vi "_CSMObj-Release.vi"(8 "Error in":errorcluster caption="Error in (no error)", 11 "CSMQ in":T1={"Requested Name"="", "Module Name"="", "Mode"=enum."Stand Alone", "Queue"=refnum, "CSM-Data"=refnum, "User Event"=refnum, "Status Change Event"=refnum, "Allowed Messages"=[], "Mode-Data"=refnum, "Group Name"="", "Exit Event"=refnum}) -> (0 "Error out":errorcluster, 1 "Group Release?":bool, 3 "CSMQ out":T1={"Requested Name"="", "Module Name"="", "Mode"=enum."Stand Alone", "Queue"=refnum, "CSM-Data"=refnum, "User Event"=refnum, "Status Change Event"=refnum, "Allowed Messages"=[], "Mode-Data"=refnum, "Group Name"="", "Exit Event"=refnum})   [LabVIEW 2020, in "Communicable State Machine.lvlib"]
uses:
  Communicable State Machine.lvlib
  _CSMObj.ctl
  Priority Queue.lvclass
  _CSM_MODE.ctl
  _CSMObj-Data.ctl
  _CSM Status Change Event Data.ctl
  _CSMObj-ModeData.ctl
  Priority Queue.lvclass/Priority Queue.ctl
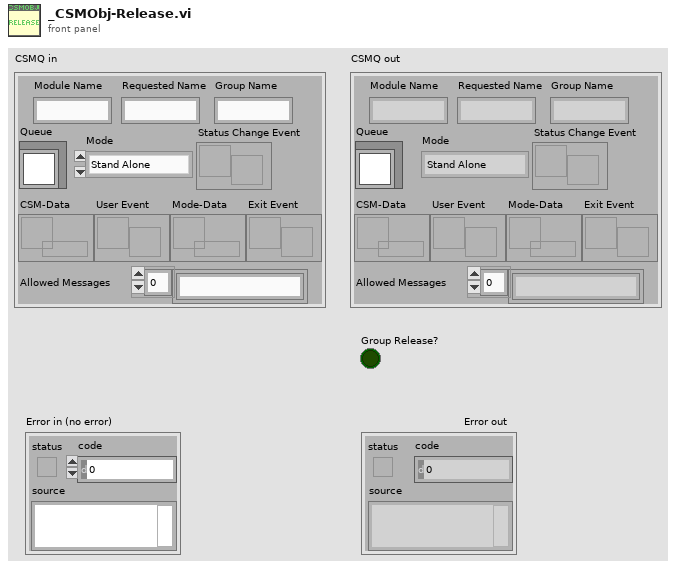
[diagram p1: front panel]
types:
  T1 = typedef "Communicable State Machine.lvlib/_CSMObj.ctl" = cluster{"Requested Name":string, "Module Name":string, "Mode":T2, "Queue":refnum<class "Priority Queue.lvclass">, "CSM-Data":refnum<data-value>, "User Event":refnum<user-event>, "Status Change Event":refnum<user-event>, "Allowed Messages":string[], "Mode-Data":refnum<data-value>, "Group Name":string, "Exit Event":refnum<user-event>}
  T2 = typedef "Communicable State Machine.lvlib/_CSM_MODE.ctl" = enum16{"Not Exist", "Stand Alone", "CSM", "Worker Agent", "Worker", "Chain", "Chain Node"}
  T3 = typedef "Communicable State Machine.lvlib/_CSMObj-ModeData.ctl" = cluster{"Share Count":i32, "Messages of Chain Nodes":cluster{"Module Name":string, "Allowed Messages":string[]}[], "Chain Message Mapping Map":variant}
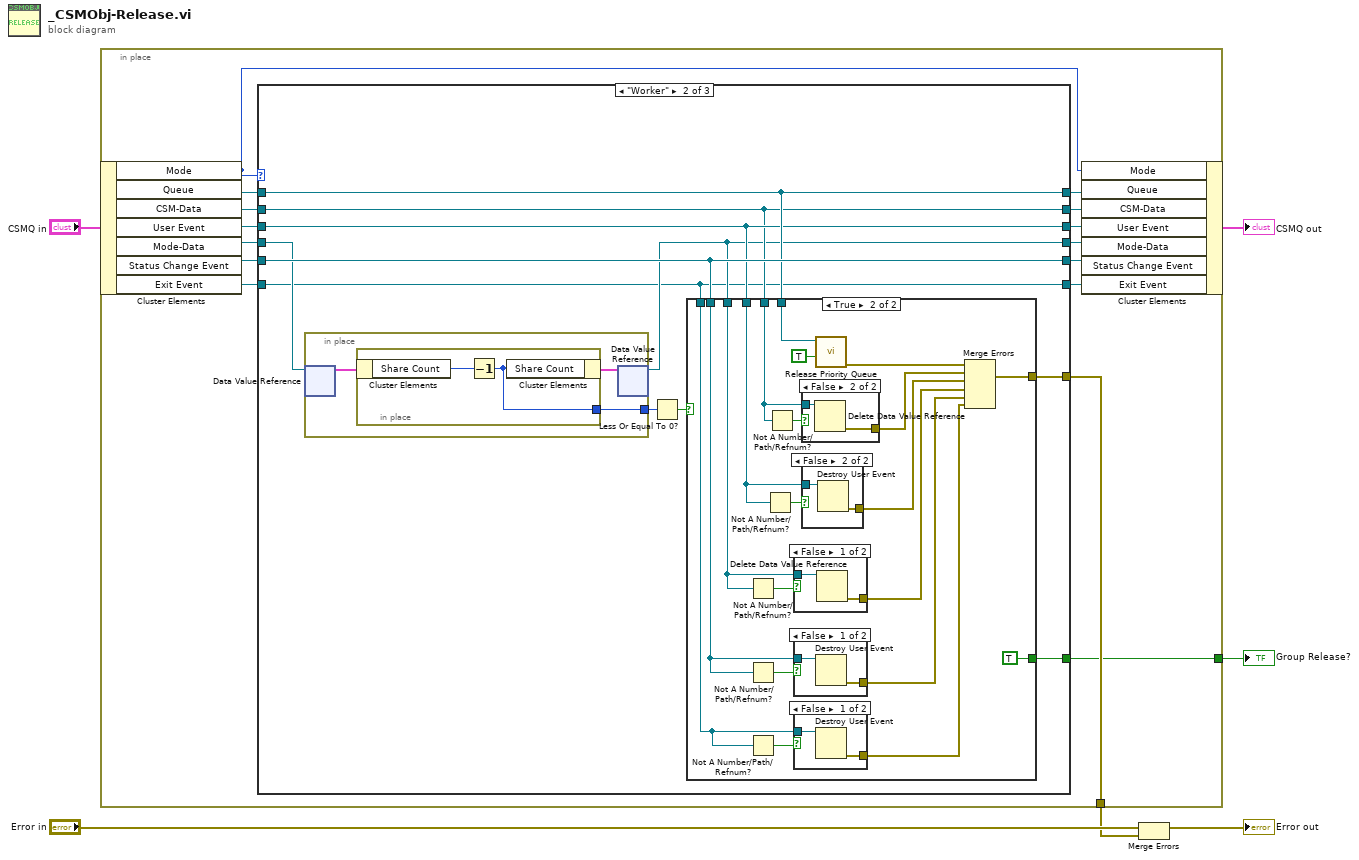
[diagram p0: block diagram]
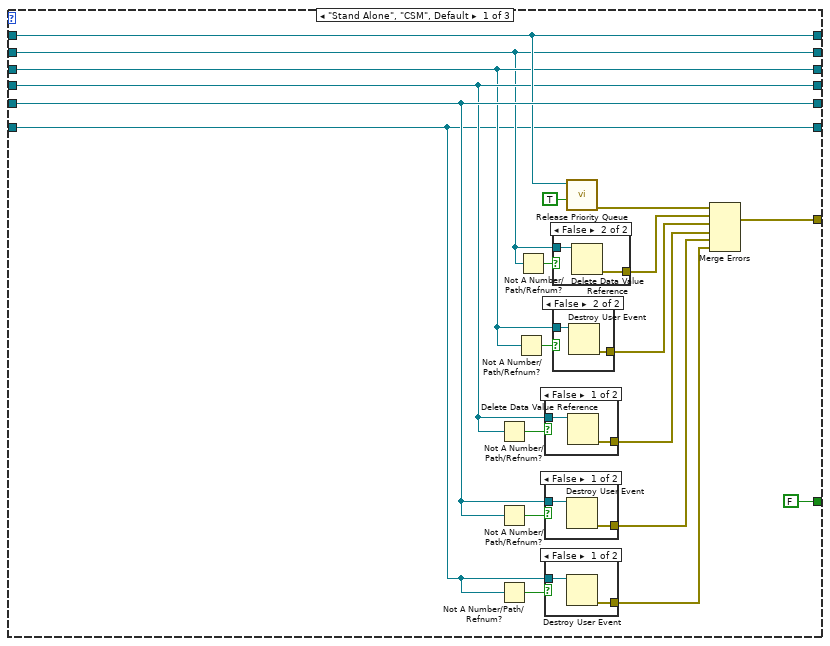
[diagram p2: hidden frame]
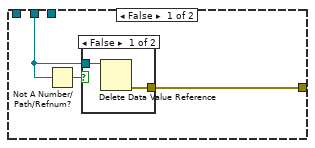
[diagram p8: hidden frame]
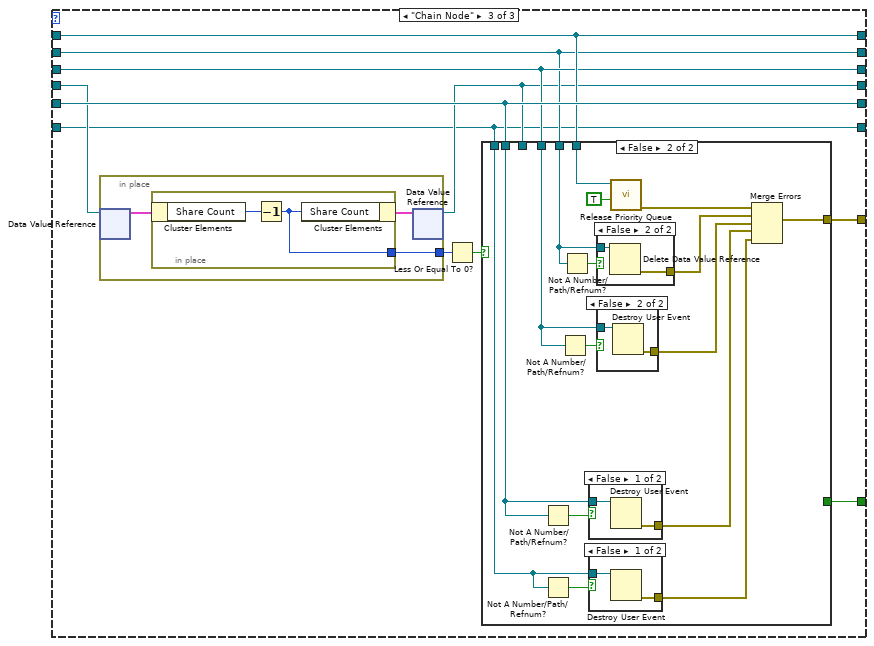
[diagram p15: hidden frame]
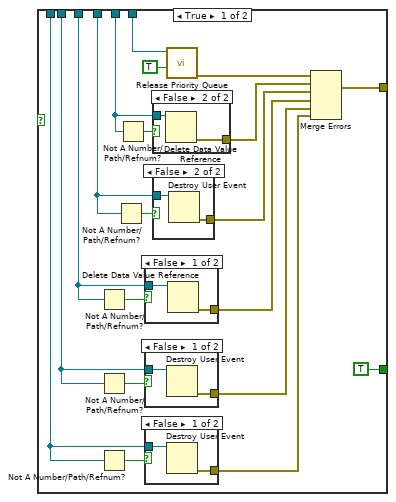
[diagram p16: hidden frame]
diagram:
  n1 = in-place "In Place Element Structure" {
    in-place-border: [w12] -> w2
    in-place-border: [w11] -> w1
    n2 = in-place-cluster #1("CSMQ in") -> ("Mode"=w9:T2, "Queue"=w17:refnum<class "Priority Queue.lvclass">, "CSM-Data"=w20:refnum<data-value>, "User Event"=w19:refnum<user-event>, "Mode-Data"=w21:refnum<data-value>, "Status Change Event"=w18:refnum<user-event>, "Exit Event"=w7:refnum<user-event>)
    n3 = case shown="\"Worker\"" w9 {
      tunnel: w21 -> [w29 w56 w107]
      tunnel: w20 -> [w26 w57 w108]
      tunnel: w19 -> [w28 w58 w109]
      tunnel: w18 -> [w41 w62 w113]
      tunnel: w17 -> [w40 w61 w112]
      tunnel: [w41 w62 w113] -> w16
      tunnel: [w28 w58 w109] -> w15
      tunnel: [w26 w57 w108] -> w14
      tunnel: [w40 w61 w112] -> w13
      tunnel: [w39 w60 w111] -> w12
      tunnel: [FALSE w59 w110] -> w11
      tunnel: [w29 w55 w106] -> w10
      tunnel: [w23 w52 w103] -> w8
      tunnel: w7 -> [w23 w52 w103]
      frame "Stand Alone", "CSM", Default {
        n4 = Not A Number/Path/Refnum?(number/path/refnum=w29) -> (NaN/Path/Refnum?=w31:bool)
        n5 = Not A Number/Path/Refnum?(number/path/refnum=w41) -> (NaN/Path/Refnum?=w32:bool)
        n6 = Not A Number/Path/Refnum?(number/path/refnum=w23) -> (NaN/Path/Refnum?=w24:bool)
        n7 = Not A Number/Path/Refnum?(number/path/refnum=w28) -> (NaN/Path/Refnum?=w27:bool)
        n8 = Not A Number/Path/Refnum?(number/path/refnum=w26) -> (NaN/Path/Refnum?=w25:bool)
        n9 = case shown="False" w31 {
          tunnel: [w49 _] -> w30
          tunnel: w29 -> [w48 _]
          frame False {
            n10 = Delete Data Value Reference(data value reference=w48) -> (error out=w49:errorcluster)  [unwired: 1 in, 1 out]
          }
          frame True {
          }
        }
        n11 = case shown="False" w32 {
          tunnel: [w51 _] -> w33
          tunnel: w41 -> [w50 _]
          frame False {
            n12 = Destroy User Event(user event=w50) -> (error out=w51:errorcluster)  [unwired: 1 in]
          }
          frame True {
          }
        }
        n13 = case shown="False" w24 {
          tunnel: [w43 _] -> w22
          tunnel: w23 -> [w42 _]
          frame False {
            n14 = Destroy User Event(user event=w42) -> (error out=w43:errorcluster)  [unwired: 1 in]
          }
          frame True {
          }
        }
        n15 = case shown="False" w25 {
          tunnel: [_ w45] -> w35
          tunnel: w26 -> [_ w44]
          frame True {
          }
          frame False {
            n16 = Delete Data Value Reference(data value reference=w44) -> (error out=w45:errorcluster)  [unwired: 1 in, 1 out]
          }
        }
        n17 = case shown="False" w27 {
          tunnel: [_ w47] -> w34
          tunnel: w28 -> [_ w46]
          frame True {
          }
          frame False {
            n18 = Destroy User Event(user event=w46) -> (error out=w47:errorcluster)  [unwired: 1 in]
          }
        }
        n19 = call "Release Priority Queue.vi"("force destroy? (F)"=TRUE, "Priority Queue"=w40) -> ("error out"=w36:errorcluster)  [unwired: 9 in]
        n20 = Merge Errors(w36, w35, w34, w30, w33, w22) -> (w39:errorcluster)
      }
      frame "Worker" {
        n21 = in-place {
          in-place-border: [w98] -> w54
          n22 = in-place-dvr #2(w56) -> (w100:T3)  [unwired: 1 out]
          n23 = in-place {
            in-place-border: [w101] -> w98
            n24 = in-place-cluster #3(w100) -> ("Share Count"=w102:i32)
            n25 = Decrement(x=w102) -> (x-1=w101:i32)
            n26 = in-place-cluster #3("Share Count"=w101) -> (w99:T3)
          }
          n27 = in-place-dvr #2(w99) -> (w55:refnum<data-value>)  [unwired: 1 out]
        }
        n28 = Less Or Equal To 0?(x=w54) -> (x <= 0?=w53:bool)
        n29 = case shown="True" w53 {
          tunnel: w62 -> [_ w87]
          tunnel: w61 -> [_ w86]
          tunnel: [w63 w85] -> w60
          tunnel: [_ TRUE] -> w59
          tunnel: w58 -> [_ w75]
          tunnel: w57 -> [w64 w73]
          tunnel: w55 -> [_ w71]
          tunnel: w52 -> [_ w69]
          frame False {
            n30 = Not A Number/Path/Refnum?(number/path/refnum=w64) -> (NaN/Path/Refnum?=w65:bool)
            n31 = case shown="False" w65 {
              tunnel: [w67 _] -> w63
              tunnel: w64 -> [w66 _]
              frame False {
                n32 = Delete Data Value Reference(data value reference=w66) -> (error out=w67:errorcluster)  [unwired: 1 in, 1 out]
              }
              frame True {
              }
            }
          }
          frame True {
            n33 = Not A Number/Path/Refnum?(number/path/refnum=w71) -> (NaN/Path/Refnum?=w77:bool)
            n34 = Not A Number/Path/Refnum?(number/path/refnum=w87) -> (NaN/Path/Refnum?=w78:bool)
            n35 = Not A Number/Path/Refnum?(number/path/refnum=w69) -> (NaN/Path/Refnum?=w70:bool)
            n36 = Not A Number/Path/Refnum?(number/path/refnum=w75) -> (NaN/Path/Refnum?=w74:bool)
            n37 = Not A Number/Path/Refnum?(number/path/refnum=w73) -> (NaN/Path/Refnum?=w72:bool)
            n38 = case shown="False" w77 {
              tunnel: [w95 _] -> w76
              tunnel: w71 -> [w94 _]
              frame False {
                n39 = Delete Data Value Reference(data value reference=w94) -> (error out=w95:errorcluster)  [unwired: 1 in, 1 out]
              }
              frame True {
              }
            }
            n40 = case shown="False" w78 {
              tunnel: [w97 _] -> w79
              tunnel: w87 -> [w96 _]
              frame False {
                n41 = Destroy User Event(user event=w96) -> (error out=w97:errorcluster)  [unwired: 1 in]
              }
              frame True {
              }
            }
            n42 = case shown="False" w70 {
              tunnel: [w89 _] -> w68
              tunnel: w69 -> [w88 _]
              frame False {
                n43 = Destroy User Event(user event=w88) -> (error out=w89:errorcluster)  [unwired: 1 in]
              }
              frame True {
              }
            }
            n44 = case shown="False" w72 {
              tunnel: [_ w91] -> w81
              tunnel: w73 -> [_ w90]
              frame True {
              }
              frame False {
                n45 = Delete Data Value Reference(data value reference=w90) -> (error out=w91:errorcluster)  [unwired: 1 in, 1 out]
              }
            }
            n46 = case shown="False" w74 {
              tunnel: [_ w93] -> w80
              tunnel: w75 -> [_ w92]
              frame True {
              }
              frame False {
                n47 = Destroy User Event(user event=w92) -> (error out=w93:errorcluster)  [unwired: 1 in]
              }
            }
            n48 = call "Release Priority Queue.vi"("force destroy? (F)"=TRUE, "Priority Queue"=w86) -> ("error out"=w82:errorcluster)  [unwired: 9 in]
            n49 = Merge Errors(w82, w81, w80, w76, w79, w68) -> (w85:errorcluster)
          }
        }
      }
      frame "Chain Node" {
        n50 = in-place {
          in-place-border: [w168] -> w105
          n51 = in-place-dvr #4(w107) -> (w170:T3)  [unwired: 1 out]
          n52 = in-place {
            in-place-border: [w171] -> w168
            n53 = in-place-cluster #5(w170) -> ("Share Count"=w172:i32)
            n54 = Decrement(x=w172) -> (x-1=w171:i32)
            n55 = in-place-cluster #5("Share Count"=w171) -> (w169:T3)
          }
          n56 = in-place-dvr #4(w169) -> (w106:refnum<data-value>)  [unwired: 1 out]
        }
        n57 = Less Or Equal To 0?(x=w105) -> (x <= 0?=w104:bool)
        n58 = case shown="False" w104 {
          tunnel: w113 -> [w133 w159]
          tunnel: w112 -> [w132 w158]
          tunnel: [w131 w157] -> w111
          tunnel: [TRUE _] -> w110
          tunnel: w109 -> [w121 w150]
          tunnel: w108 -> [w119 w148]
          tunnel: w106 -> [w117 _]
          tunnel: w103 -> [w115 w145]
          frame True {
            n59 = Not A Number/Path/Refnum?(number/path/refnum=w117) -> (NaN/Path/Refnum?=w123:bool)
            n60 = Not A Number/Path/Refnum?(number/path/refnum=w133) -> (NaN/Path/Refnum?=w124:bool)
            n61 = Not A Number/Path/Refnum?(number/path/refnum=w115) -> (NaN/Path/Refnum?=w116:bool)
            n62 = Not A Number/Path/Refnum?(number/path/refnum=w121) -> (NaN/Path/Refnum?=w120:bool)
            n63 = Not A Number/Path/Refnum?(number/path/refnum=w119) -> (NaN/Path/Refnum?=w118:bool)
            n64 = case shown="False" w123 {
              tunnel: [w141 _] -> w122
              tunnel: w117 -> [w140 _]
              frame False {
                n65 = Delete Data Value Reference(data value reference=w140) -> (error out=w141:errorcluster)  [unwired: 1 in, 1 out]
              }
              frame True {
              }
            }
            n66 = case shown="False" w124 {
              tunnel: [w143 _] -> w125
              tunnel: w133 -> [w142 _]
              frame False {
                n67 = Destroy User Event(user event=w142) -> (error out=w143:errorcluster)  [unwired: 1 in]
              }
              frame True {
              }
            }
            n68 = case shown="False" w116 {
              tunnel: [w135 _] -> w114
              tunnel: w115 -> [w134 _]
              frame False {
                n69 = Destroy User Event(user event=w134) -> (error out=w135:errorcluster)  [unwired: 1 in]
              }
              frame True {
              }
            }
            n70 = case shown="False" w118 {
              tunnel: [_ w137] -> w127
              tunnel: w119 -> [_ w136]
              frame True {
              }
              frame False {
                n71 = Delete Data Value Reference(data value reference=w136) -> (error out=w137:errorcluster)  [unwired: 1 in, 1 out]
              }
            }
            n72 = case shown="False" w120 {
              tunnel: [_ w139] -> w126
              tunnel: w121 -> [_ w138]
              frame True {
              }
              frame False {
                n73 = Destroy User Event(user event=w138) -> (error out=w139:errorcluster)  [unwired: 1 in]
              }
            }
            n74 = call "Release Priority Queue.vi"("force destroy? (F)"=TRUE, "Priority Queue"=w132) -> ("error out"=w128:errorcluster)  [unwired: 9 in]
            n75 = Merge Errors(w128, w127, w126, w122, w125, w114) -> (w131:errorcluster)
          }
          frame False {
            n76 = Not A Number/Path/Refnum?(number/path/refnum=w159) -> (NaN/Path/Refnum?=w151:bool)
            n77 = Not A Number/Path/Refnum?(number/path/refnum=w145) -> (NaN/Path/Refnum?=w146:bool)
            n78 = Not A Number/Path/Refnum?(number/path/refnum=w150) -> (NaN/Path/Refnum?=w149:bool)
            n79 = Not A Number/Path/Refnum?(number/path/refnum=w148) -> (NaN/Path/Refnum?=w147:bool)
            n80 = case shown="False" w151 {
              tunnel: [w167 _] -> w152
              tunnel: w159 -> [w166 _]
              frame False {
                n81 = Destroy User Event(user event=w166) -> (error out=w167:errorcluster)  [unwired: 1 in]
              }
              frame True {
              }
            }
            n82 = case shown="False" w146 {
              tunnel: [w161 _] -> w144
              tunnel: w145 -> [w160 _]
              frame False {
                n83 = Destroy User Event(user event=w160) -> (error out=w161:errorcluster)  [unwired: 1 in]
              }
              frame True {
              }
            }
            n84 = case shown="False" w147 {
              tunnel: [_ w163] -> w154
              tunnel: w148 -> [_ w162]
              frame True {
              }
              frame False {
                n85 = Delete Data Value Reference(data value reference=w162) -> (error out=w163:errorcluster)  [unwired: 1 in, 1 out]
              }
            }
            n86 = case shown="False" w149 {
              tunnel: [_ w165] -> w153
              tunnel: w150 -> [_ w164]
              frame True {
              }
              frame False {
                n87 = Destroy User Event(user event=w164) -> (error out=w165:errorcluster)  [unwired: 1 in]
              }
            }
            n88 = call "Release Priority Queue.vi"("force destroy? (F)"=TRUE, "Priority Queue"=w158) -> ("error out"=w155:errorcluster)  [unwired: 9 in]
            n89 = Merge Errors(w155, w154, w153, w152, w144) -> (w157:errorcluster)
          }
        }
      }
    }
    n90 = in-place-cluster #1("Mode"=w9, "Queue"=w13, "CSM-Data"=w14, "User Event"=w15, "Mode-Data"=w10, "Status Change Event"=w16, "Exit Event"=w8) -> (→"CSMQ out":T1)
  }
  "Group Release?" <- w1
  n91 = Merge Errors("Error in", w2) -> (→"Error out":errorcluster)
